vi "sensor efecto hall.vi"() -> ()   [LabVIEW 2016]
uses:
  <vilib>/MakerHub/LINX/Public/Peripherals/Analog/Analog Read 1 Chan.vi
  <vilib>/MakerHub/LINX/Public/Peripherals/Digital/Digital Read 1 Chan.vi
  <vilib>/MakerHub/LINX/Public/Peripherals/Digital/Digital Write 1 Chan.vi
  <vilib>/MakerHub/LINX/Public/Peripherals/Analog/Analog Read N Chans.vi
  <vilib>/MakerHub/LINX/Public/Peripherals/Digital/Digital Read N Chans.vi
  <vilib>/MakerHub/LINX/Public/Peripherals/Digital/Digital Write N Chans.vi
  <vilib>/MakerHub/LINX/Private/Local IO/LinxAnalogRead.vi
  <vilib>/MakerHub/LINX/Public/Utilities/Check Channel.vi
  <vilib>/MakerHub/LINX/Private/Local IO/LinxDigitalRead.vi
  <vilib>/MakerHub/LINX/Private/Local IO/LinxDigitalWrite.vi
  <vilib>/MakerHub/LINX/Public/Utilities/Open Serial.vi
  <vilib>/MakerHub/LINX/Private/Utilties/Generate Error.vi
  <vilib>/MakerHub/LINX/LMH-LINX.lvlib
panel:
  in  "stop":bool
  out "Led":bool
  out "intensisdad":dbl(knob) scale=0.0..5.0
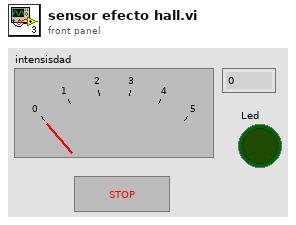
[diagram p1: front panel]
types:
  T1 = typedef "LMH-LINX.lvlib/LINX Ref.ctl" = cluster{"IO":T2, "Interface":T3, "LINX Device Config":T4}
  T2 = typedef "LMH-LINX.lvlib/Platform.ctl" = enum16{"Remote", "Local"}
  T3 = typedef "LMH-LINX.lvlib/Interface.ctl" = enum16{"Serial", "TCP"}
  T4 = typedef "LMH-LINX.lvlib/Device.lvlib/LINX Device Config.ctl" = cluster{"Interface":T3, "COM Port":refnum<visa-resource-name>, "TCP Configuration":T5, "Device Family":u8, "Device ID":u8, "Device Name":string, "TCP Ref":refnum<k5>, "Channels":T6}
  T5 = typedef "LMH-LINX.lvlib/Device.lvlib/TCP Config.ctl" = cluster{"IP Address":string, "Port":u16}
  T6 = typedef "LMH-LINX.lvlib/Channels.ctl" = cluster{"DI":u8[], "DO":u8[], "AI":u8[], "AO":u8[], "PWM":u8[], "QE":u8[], "UART":u8[], "I2C 2":u8[], "SPI":u8[], "CAN":u8[], "Servo":u8[], "AI Ref (V)":dbl, "AI Resolution (Bits)":u8, "AO Ref (V)":dbl, "AO Resolution (Bits)":u8}
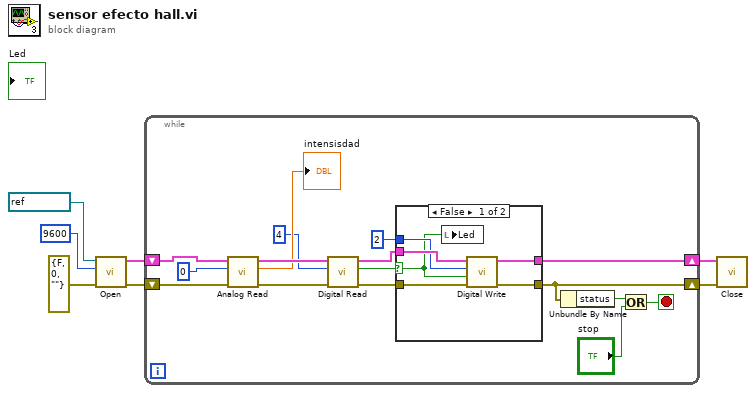
[diagram p0: block diagram]
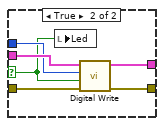
[diagram p2: hidden frame]
diagram:
  n1 = call-poly <vilib>:"Open.vi"("Error In"=errorcluster {"status"=FALSE, "code"=0, "source"=""}, "Baud Rate Override"=u32 9600, "Serial Port"=refnum<visa-resource-name> "COM6") -> ("Error Out"=w3:errorcluster, "LINX Resource"=w4:T1)  [unwired: 6 in, 1 out]
  n2 = while {
    shift-right: [w10] -> w2
    shift-left: w4 -> [w22]
    shift-right: [w8] -> w1
    shift-left: w3 -> [w21]
    stop <- w11 stop-if-true
    n3 = call-poly <vilib>:"Analog Read.vi"("Error In"=w21, "Analog Channel"=u8 0, "LINX Resource"=w22) -> ("Error Out"=w19:errorcluster, "Voltage"=→"intensisdad":dbl, "LINX Resource"=w20:T1)  [unwired: 5 in, 1 out]
    n4 = call-poly <vilib>:"Digital Read.vi"("Error In"=w19, "DI Channel"=u8 4, "LINX Resource"=w20) -> ("Error Out"=w14:errorcluster, "DI Value"=w16:bool, "LINX Resource"=w15:T1)  [unwired: 6 in]
    n5 = case shown="False" w16 {
      selector: w16 -> [w24 w30]
      tunnel: w15 -> [w29 w35]
      tunnel: w14 -> [w28 w33]
      tunnel: u8 2 ("DI Channel") -> [w27 w34]
      tunnel: [w26 w32] -> w10
      tunnel: [w25 w31] -> w8
      frame False {
        n6 = local write "Led"(w24) -> ()
        n7 = call-poly <vilib>:"Digital Write.vi"("Error In"=w28, "Output Value"=w24, "DO Channel"=w27, "LINX Resource"=w29) -> ("Error Out"=w25:errorcluster, "LINX Resource"=w26:T1)  [unwired: 6 in]
      }
      frame True {
        n8 = local write "Led"(w30) -> ()
        n9 = call-poly <vilib>:"Digital Write.vi"("Error In"=w33, "Output Value"=w30, "DO Channel"=w34, "LINX Resource"=w35) -> ("Error Out"=w31:errorcluster, "LINX Resource"=w32:T1)  [unwired: 6 in]
      }
    }
    n10 = Unbundle By Name(w8) -> ("status"=w9:bool)
    n11 = Or(x=w9, y="stop") -> (x .or. y?=w11:bool)
  }
  n12 = call <vilib>:"Close.vi"("Error In"=w1, "LINX Resource"=w2) -> ()  [unwired: 9 in, 1 out]
